vi "Write Abort String.vi"(8 "Helium Fail":i32[](array[numeric]), 9 "Vacuum Fail":i32[](array[numeric]), 10 "Test Results":T1, 11 "Summary In":string[](array[string])) -> (1 "Summary Out":string[][](array[string]))   [LabVIEW 2014]
uses:
  Tests/Controls/Test Results.ctl
  Tests/Controls/Step Result.ctl
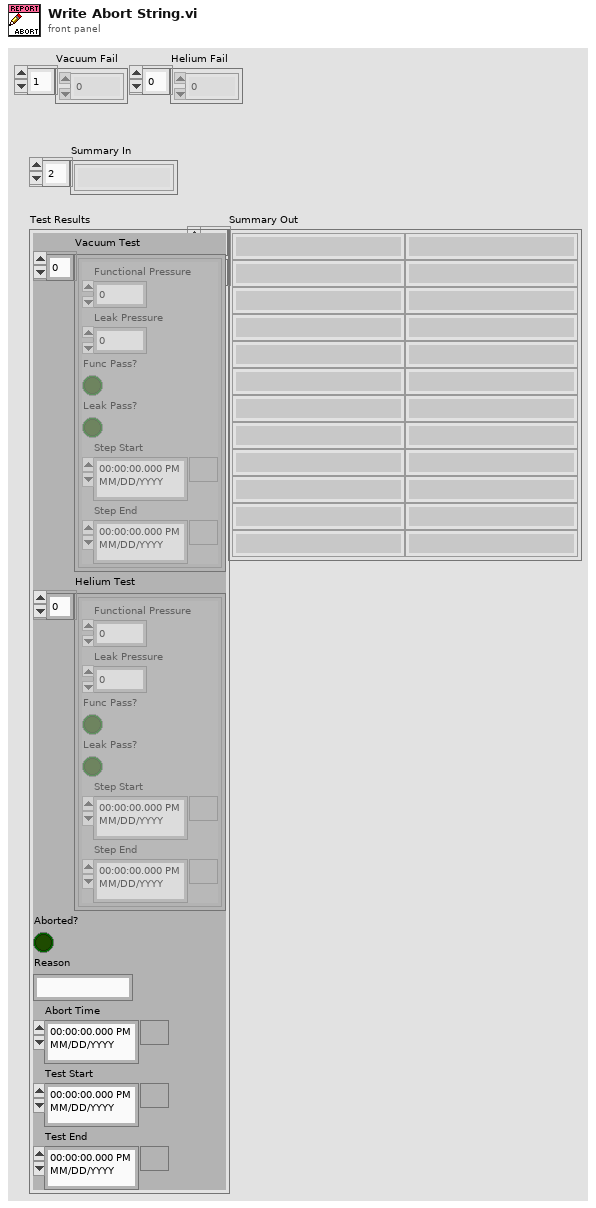
[diagram p1: front panel]
types:
  T1 = typedef "Test Results.ctl" = cluster{"Vacuum Test":T2[], "Helium Test":T2[], "Aborted?":bool, "Reason":string, "Abort Time":timestamp, "Test Start":timestamp, "Test End":timestamp}
  T2 = typedef "Step Result.ctl" = cluster{"Functional Pressure":dbl, "Leak Pressure":dbl, "Func Pass?":bool, "Leak Pass?":bool, "Step Start":timestamp, "Step End":timestamp}
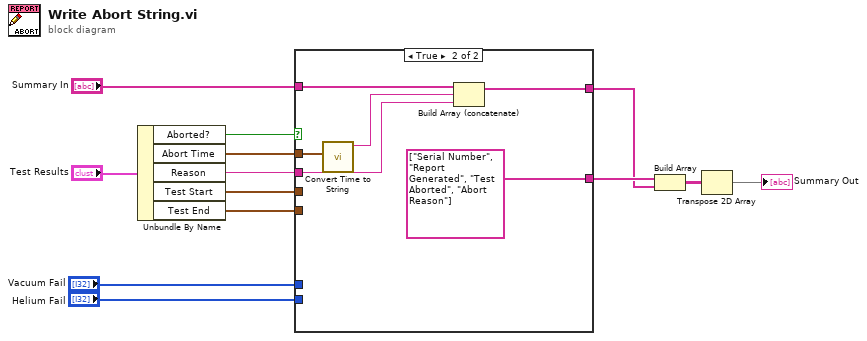
[diagram p0: block diagram]
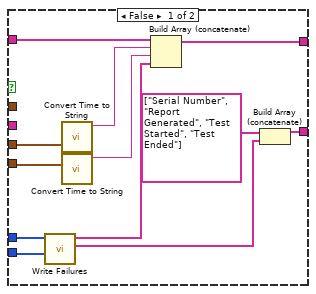
[diagram p2: hidden frame]
diagram:
  n1 = Unbundle By Name("Test Results") -> ("Aborted?"=w9:bool, "Abort Time"=w11:timestamp, "Reason"=w12:string, "Test Start"=w7:timestamp, "Test End"=w6:timestamp)
  n2 = case shown="True" w9 {
    tunnel: "Summary In" -> [w20 w31]
    tunnel: w11 -> [_ w29]
    tunnel: w12 -> [_ w27]
    tunnel: [w23 w30] -> w3
    tunnel: [w14 string[] ["Serial Number", "Report Generated", "Test Aborted", "Abort Reason"] ("Abort")] -> w4
    tunnel: w7 -> [w25 _]
    tunnel: w6 -> [w24 _]
    tunnel: "Vacuum Fail" -> [w19 _]
    tunnel: "Helium Fail" -> [w18 _]
    frame False {
      n3 = call "Write Failures.vi"("Helium Fail"=w18, "Vacuum Fail"=w19) -> ("Headers"=w15:string[], "Failures"=w17:string[])  [unwired: 8 in]
      n4 = call "Convert Time to String.vi"("time stamp"=w25) -> ("date/time string"=w22:string)  [unwired: 10 in]
      n5 = call "Convert Time to String.vi"("time stamp"=w24) -> ("date/time string"=w21:string)  [unwired: 10 in]
      n6 = Build Array (concatenate)(w20, w22, w21, w17) -> (w23:string[])
      n7 = Build Array (concatenate)(string[] ["Serial Number", "Report Generated", "Test Started", "Test Ended"] ("Success"), w15) -> (w14:string[])
    }
    frame True {
      n8 = call "Convert Time to String.vi"("time stamp"=w29) -> ("date/time string"=w28:string)  [unwired: 10 in]
      n9 = Build Array (concatenate)(w31, w28, w27) -> (w30:string[])
    }
  }
  n10 = Build Array(w4, w3) -> (w13:string[][])
  n11 = Transpose 2D Array(2D array=w13) -> (transposed array=→"Summary Out":string[][])
